vi "ConvertTimeStampFormatLvToDb.vi"(10 "to UTC (F)":bool=TRUE, 11 "Time Stamp":timestamp) -> (3 "output string":string)   [LabVIEW 2019]
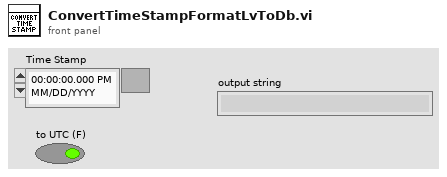
[diagram p1: front panel]
types:
  T1 = typedef "LVDateTimeRec.ctl" = cluster{"fractional second":dbl, "second":i32, "minute":i32, "hour":i32, "day of month":i32, "month":i32, "year":i32, "day of week":i32, "day of year":i32, "DST":i32}
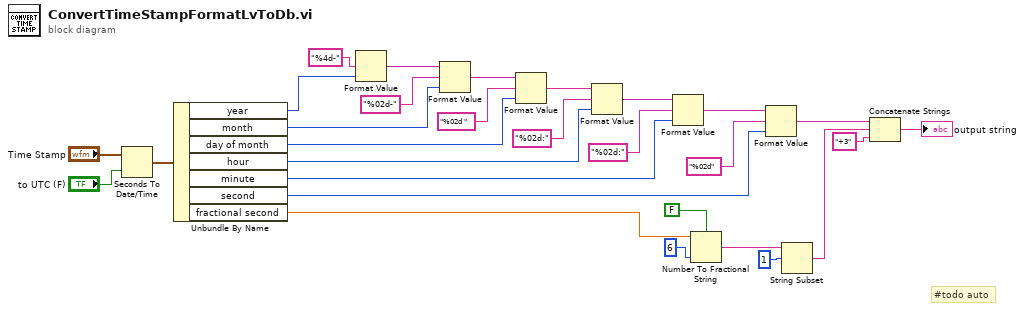
[diagram p0: block diagram]
diagram:
  # "#todo auto"
  n1 = Seconds To Date/Time(time stamp (now)="Time Stamp", to UTC (F)="to UTC (F)") -> (date time rec=w10:T1)
  n2 = Unbundle By Name(w10) -> ("year"=w25:i32, "month"=w26:i32, "day of month"=w17:i32, "hour"=w19:i32, "minute"=w18:i32, "second"=w20:i32, "fractional second"=w8:dbl)
  n3 = Format Value(format string="%4d-", value (0)=w25) -> (output string=w11:string)  [unwired: 1 out]
  n4 = Format Value(string ("")=w11, format string="%02d-", value (0)=w26) -> (output string=w12:string)
  n5 = Format Value(string ("")=w12, format string="%02d ", value (0)=w17) -> (output string=w13:string)
  n6 = Format Value(string ("")=w13, format string="%02d:", value (0)=w19) -> (output string=w14:string)
  n7 = Format Value(string ("")=w14, format string="%02d:", value (0)=w18) -> (output string=w15:string)
  n8 = Number To Fractional String(use system decimal point (T)=FALSE, number=w8, precision (6)=i16 6) -> (F-format string=w5:string)  [unwired: 1 in]
  n9 = Format Value(string ("")=w15, format string="%02d", value (0)=w20) -> (output string=w9:string)
  n10 = String Subset(string=w5, offset (0)=1) -> (substring=w2:string)  [unwired: 1 in]
  n11 = Concatenate Strings(w9, w2, "+3" ("string")) -> (→"output string":string)
